vi "getDataAsTable.vi"(8 "error in (no error)":errorcluster, 11 "TransactionList in":refnum<class "TransactionList.lvclass">) -> (0 "error out":errorcluster, 2 "Table Row":string[][](array[string]), 3 "TransactionList out":refnum<class "TransactionList.lvclass">)   [LabVIEW 2018, in "TransactionList.lvclass"]
uses:
  TransactionList.lvclass
  TransactionList.lvclass/TransactionList.ctl
  Transaction/Transaction.lvclass
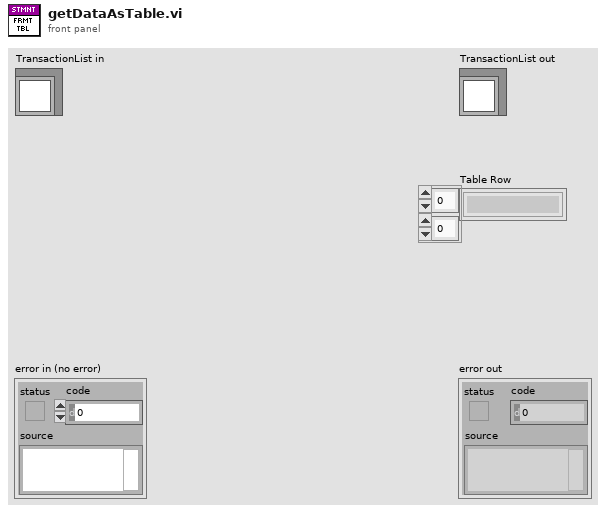
[diagram p1: front panel]
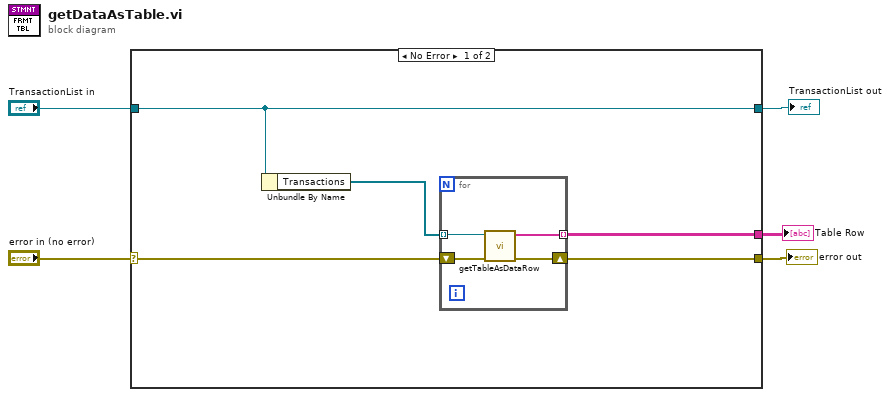
[diagram p0: block diagram]
diagram:
  n1 = case shown="No Error" "error in (no error)" {
    selector: "error in (no error)" -> [w6 w16]
    tunnel: [w10 w16] -> w4
    tunnel: [w8 w15] -> w2
    tunnel: "TransactionList in" -> [w8 w15]
    tunnel: [w9 _] -> w1
    frame No Error {
      n2 = Unbundle By Name(w8) -> ("Transactions"=w7:refnum<class "Transaction.lvclass">[])
      n3 = for {
        tunnel: w7 -> [w14] mode=indexing
        tunnel: [w13] -> w9 mode=indexing
        shift-right: [w11] -> w10
        shift-left: w6 -> [w12]
        n4 = call "getTableAsDataRow.vi"("error in (no error)"=w12, "Transaction in"=w14) -> ("error out"=w11:errorcluster, "Table Row"=w13:string[])  [unwired: 8 in]
      }
    }
    frame Error {
    }
  }
  "error out" <- w4
  "TransactionList out" <- w2
  "Table Row" <- w1
